vi "Untitled 1.vi"() -> ()   [LabVIEW 2019]
uses:
  <vilib>/vision/NI_Vision_Development_Module.lvlib
panel:
  out "Image":T1(plugin-control)
  in  "File Path":path
  out "Ellipses":T2(array[cluster]) {"Position"."Y" format="%.2f"; "Position"."X" format="%.2f"}
  out "Number of Matches Returned":i32
  in  "stop":bool
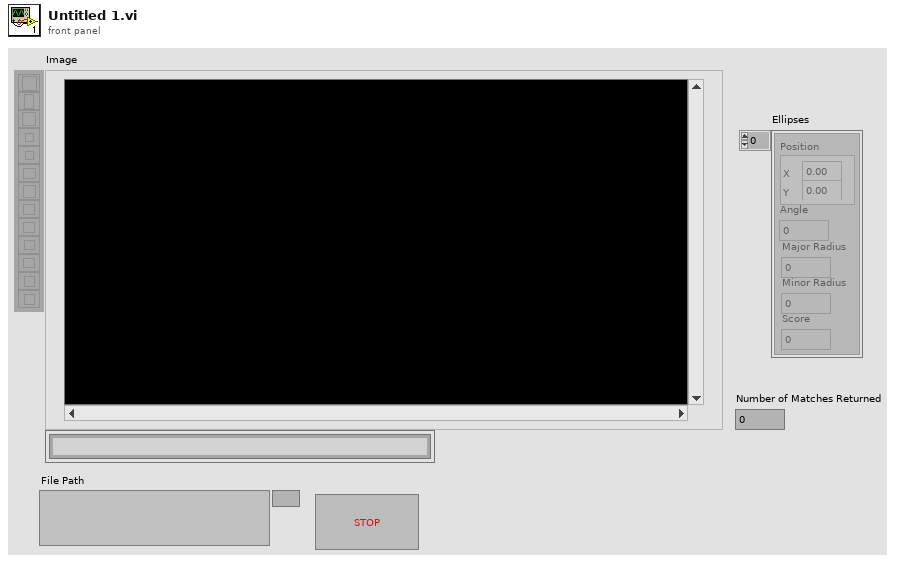
[diagram p1: front panel]
types:
  T1 = typedef "IMAQ Image.ctl" = refnum<image>
  T2 = cluster{"Position":cluster{"X":sgl, "Y":sgl}, "Angle":dbl, "Major Radius":dbl, "Minor Radius":dbl, "Score":dbl}[]
  T3 = cluster{"Global Rectangle":i32[], "Contours":cluster{"Contour Type":u32, "ROI Type":u32, "Points":i32[]}[]}
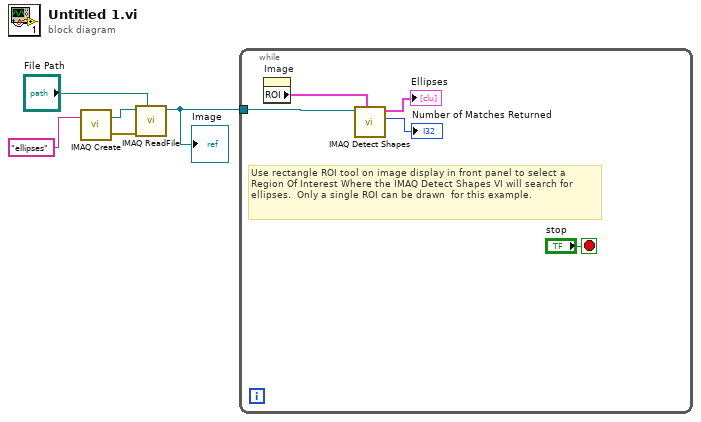
[diagram p0: block diagram]
diagram:
  n1 = call "IMAQ Create"("Image Name"="ellipses") -> ("New Image"=w2:T1, "error out"=w1:errorcluster)  [unwired: 4 in]
  n2 = call "IMAQ ReadFile"("File Path"="File Path", "error in (no error)"=w1, "Image"=w2) -> ("Image Out"=w5:T1)  [unwired: 4 in, 4 out]
  "Image" <- w5
  n3 = while {
    tunnel: w5 -> [w9]
    stop <- "stop" stop-if-true
    # "Use rectangle ROI tool on image display in front panel to select a Region Of Interest Where the IMAQ Detect Shapes VI will search for ellipses.  Only a single ROI can be drawn  for this example."
    n4 = property on="Image" class="ImageControl"() -> ("ROI"=w6:T3)  [unwired: 2 in, 2 out]
    n5 = call-poly "IMAQ Detect Shapes"("ROI Descriptor"=w6, "Image"=w9) -> ("Number of Matches Returned"=→"Number of Matches Returned":i32, "Ellipses"=→"Ellipses":T2)  [unwired: 7 in, 1 out]
  }
